vi "ManualOverrideOCU.vi"() -> ()   [LabVIEW 2011]
doc: "The Manual Override, first and foremost, allows the user to switch the boat from autonomous to override from the front panel. It's secondary function is to control the boat with keys. Currently the arrow keys connect to the sail, and the WASD keys connect to the rudder, as shown in the front panel labels. It is clearly illustrated how the keys change the value and then which values are sent to the global. You can easily change which keys do what by going to the back panel and changing the key tests.\n\nCreated by Eric Jones and Eric Schneider"
uses:
  2-Think/2 Typedefs/setpoints to boat.ctl
  2-Think/2 Typedefs/sail setpt.ctl
  2-Think/2 Typedefs/rudder angle.ctl
  2-Think/2 Typedefs/manual override.ctl
  2-Think/2 Globals/2 Global.vi
panel:
  in  "OVERRIDE?":bool
  in  "VI stop":bool
  out "Sent Rudder Angle":dbl(slide) scale=-30.0..30.0
  out "Sent Sail Value":dbl(slide) scale=0.0..1.0
  # "The Manual Override, first and foremost, allows the user to switch the boat from autonomous to override from the  front panel. It's secondary function is to control the boat with keys. Currently the arrow keys connect to the sail, and the ASDFG keys connect to the rudder, as shown in the front panel labels. It is clearly illustrated how the keys change the value and then which values are sent to the global. You can easily change which keys do what by going to the back panel and changing the key tests.\n\nToDo:\nPossibly implement a \"smart sails\" option that would allow the controller to only need to control the rudder and sails would be controlled by the boat based on heading, rudder angle, and apparent wind."
  # "SENT VALUES"
  # "SAIL CONTROL"
  # "Full Out = RIGHT"
  # "OUT = 1"
  # "Out = UP"
  # "In = DOWN"
  # "Full In = LEFT"
  # "IN = 0"
  # "RUDDER CONTROL"
  # "Full \nStarboard"
  # "Full \nPort"
  # "<--"
  # "Straight"
  # "-->"
  # "A"
  # "F"
  # "G"
  # "PORT = -30"
  # "STARB = 30"
  # "S"
  # "D"
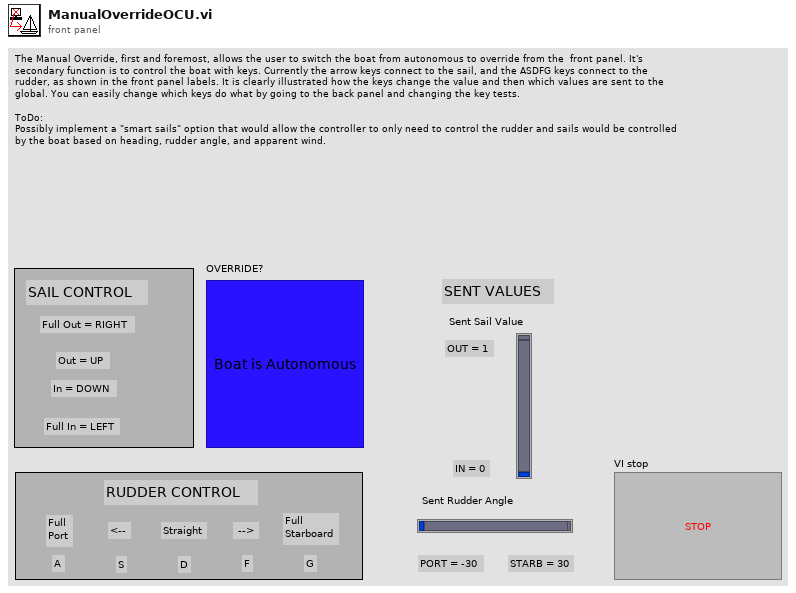
[diagram p1: front panel]
types:
  T1 = typedef "setpoints to boat.ctl" = cluster{"Sail Position":T2, "Rudder Angle":T3}
  T2 = typedef "sail setpt.ctl" = dbl
  T3 = typedef "rudder angle.ctl" = dbl
  T4 = typedef "manual override.ctl" = cluster{"Override Active":bool, "Setpoints":T1}
  T5 = typedef "eventvkey.ctl" = enum16{"ASCII", "Enter", "Return", "Shift", "Ctrl", "Alt", "Cmd", "Opt", "Caps", "NumLock", "Clear", "Break", "Up", "Down", "Left", "Right", "Insert", "Delete", "Home", "End", "PageUp", "PageDown", "Escape", "Help", "Pause", "ScrollLock", "F1", "F2", "F3", "F4", "F5", "F6", "F7", "F8", "F9", "F10", "F11", "F12", "F13", "F14", "F15", "F16", "F17", "F18", "F19", "F20", "F21", "F22", "F23", "F24", "Play", "VolumeUp", "VolumeDown", "Mute", "Two Byte Char"}
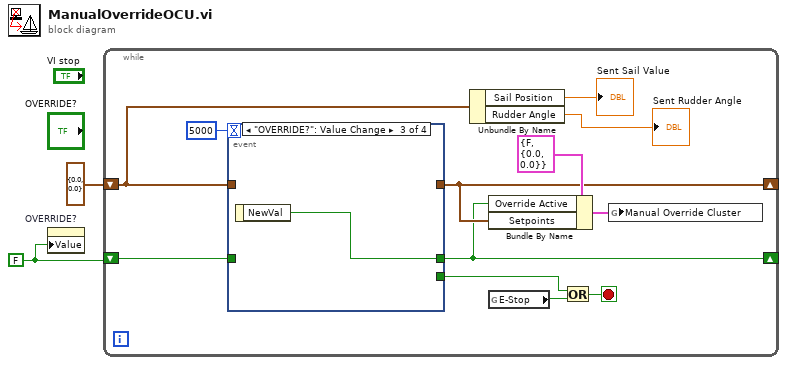
[diagram p0: block diagram]
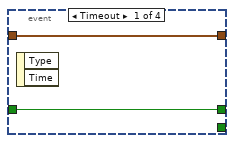
[diagram p2: hidden frame]
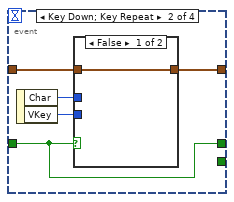
[diagram p3: hidden frame]
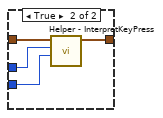
[diagram p4: hidden frame]
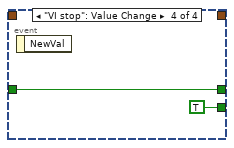
[diagram p5: hidden frame]
diagram:
  w1 = FALSE ("OVERRIDE?")
  n1 = property on="OVERRIDE?" class="Bool (strict)"("Value"=w1) -> ()  [unwired: 2 in, 2 out]
  n2 = while {
    shift-right: [w5] -> _
    shift-left: T1 {"Sail Position"=0.0, "Rudder Angle"=0.0} -> [w3]
    shift-right: [w4] -> _
    shift-left: w1 -> [w8]
    stop <- w14 stop-if-true
    n3 = event shown="[2] \"OVERRIDE?\": Value Change" {
      selector: _ -> [_ _ _ _]
      dyn-events: _ -> [_ _ _ _]
      timeout: 5000 -> [_ _ _ _]
      tunnel: w3 -> [w16 w21 _ _]
      tunnel: [w16 w20 _ _] -> w5
      tunnel: w8 -> [w15 w17 _ w28]
      tunnel: [w15 w17 w27 w28] -> w4
      tunnel: [_ _ _ TRUE ("x")] -> w6
      event Timeout {
        n4 = event-data() -> ()  [unwired: 1 in, 2 out]
      }
      event Key Down; Key Repeat {
        n5 = event-data() -> ("Char"=w19:i16, "VKey"=w18:T5)  [unwired: 1 in]
        n6 = case shown="False" w17 {
          tunnel: w21 -> [w22 w26]
          tunnel: [w22 w25] -> w20
          tunnel: w19 -> [_ w24]
          tunnel: w18 -> [_ w23]
          frame False {
          }
          frame True {
            n7 = call "Helper - InterpretKeyPress.vi"("VKey"=w23, "Char"=w24, "Command In"=w26) -> ("Command Out"=w25:T1)  [unwired: 8 in]
          }
        }
      }
      event "OVERRIDE?": Value Change {
        n8 = event-data() -> ("NewVal"=w27:bool)  [unwired: 1 in]
      }
      event "VI stop": Value Change {
        n9 = event-data() -> ()  [unwired: 1 in, 1 out]
      }
    }
    n10 = Unbundle By Name(w3) -> ("Sail Position"=→"Sent Sail Value":T2, "Rudder Angle"=→"Sent Rudder Angle":T3)
    n11 = Bundle By Name(cluster=T4 {"Override Active"=FALSE, "Setpoints"={"Sail Position"=0.0, "Rudder Angle"=0.0}}, "Override Active"=w4, "Setpoints"=w5) -> (w12:T4)
    n12 = global read "2 Global.vi" "E-Stop"() -> (w7:bool)
    n13 = Or(x=w6, y=w7) -> (x .or. y?=w14:bool)
    n14 = global write "2 Global.vi" "Manual Override Cluster"(w12) -> ()
  }
